vi "AusgabeTabelle zusammenbauen.vi"(8 "error in (no error)":errorcluster caption="Fehler (Eingang, kein Fehler)", 11 "Eingabetabelle":T2) -> (0 "error out":errorcluster caption="Fehler (Ausgang)", 1 "Eingabetabelle behandelt":string[][](array[string]), 3 "Ausgabetabelle":T1)   [LabVIEW 2020, in "Linearisierung v2.lvlib"]
uses:
  Linearisierung v2.lvlib
  Eingabetabelle.ctl
  Ausgabetabelle.ctl
panel:
  # "Tabelle:\n0.....Sollwert\n1.....Istwert\n2.....Rohwert\n3.....linearisiert\n4.....abs.Fehler ppm\n5.....Fehler in %\n6.....Deviation\n7.....Temp.Messzelle\n8.....Druck Messzelle\n9.....abs.Fehler ppm linearisiert\n10....Fehler in % linearisiert"
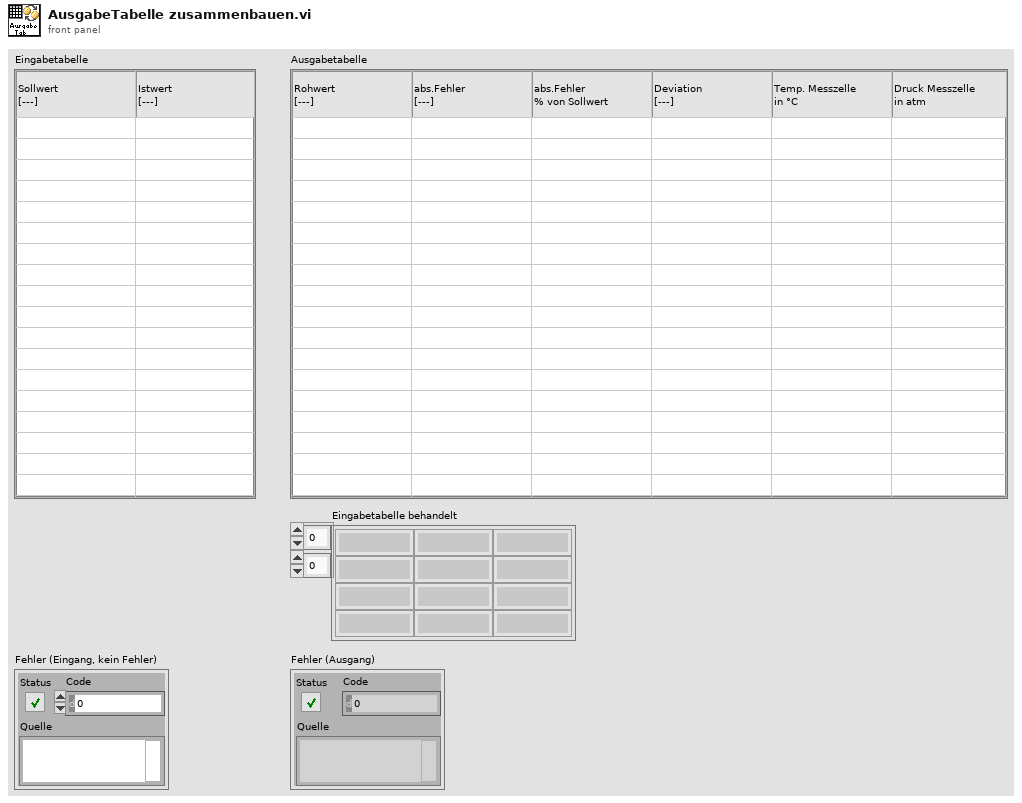
[diagram p1: front panel]
types:
  T1 = typedef "Linearisierung v2.lvlib/Ausgabetabelle.ctl" = string[][]
  T2 = typedef "Linearisierung v2.lvlib/Eingabetabelle.ctl" = string[][]
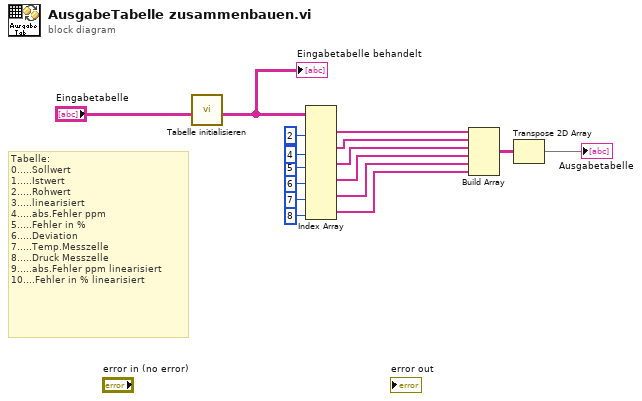
[diagram p0: block diagram]
diagram:
  # "Tabelle:\n0.....Sollwert\n1.....Istwert\n2.....Rohwert\n3.....linearisiert\n4.....abs.Fehler ppm\n5.....Fehler in %\n6.....Deviation\n7.....Temp.Messzelle\n8.....Druck Messzelle\n9.....abs.Fehler ppm linearisiert\n10....Fehler in % linearisiert"
  n1 = call "Tabelle initialisieren.vi"("Neue Tabelle"="Eingabetabelle") -> ("Tabelle"=w1:string[][])  [unwired: 10 in]
  "Eingabetabelle behandelt" <- w1
  n2 = Index Array(array=w1, index (col) #1=2 ("Deaktivierter Index (Spalte)"), index (col) #2=4 ("Index (Spalte)"), index (col) #3=5 ("Index (Spalte)"), index (col) #4=6 ("Index (Spalte)"), index (col) #5=7 ("Index (Spalte)"), index (col) #6=8 ("Index (Spalte)")) -> (element #1=w16:string[], element #2=w15:string[], element #3=w11:string[], element #4=w8:string[], element #5=w7:string[], element #6=w5:string[])  [unwired: 6 in]
  n3 = Build Array(w16, w15, w11, w8, w7, w5) -> (w4:string[][])
  n4 = Transpose 2D Array(2D array=w4) -> (transposed array=→"Ausgabetabelle":string[][])
